vi "imageAverage.vi"(0 "Camera in":refnum<class "Camera.lvclass">, 5 "data_format":T2(ring)=enum."Mono16", 7 "roi":cluster{"x0":u64, "y0":u64, "x1":u64, "y1":u64}={"x0"=18446744073709551615, "y0"=18446744073709551615, "x1"=18446744073709551615, "y1"=18446744073709551615}, 11 "error in (no error)":errorcluster) -> (4 "Camera out":refnum<class "Camera.lvclass">, 6 "image (U8)":u8[][](array[numeric]), 8 "image (U32)":u32[][](array[numeric]), 10 "image (U64)":T1(array[cluster]), 14 "raw_image (U16)":u16[][](array[numeric]), 15 "error out":errorcluster)   [LabVIEW 2019, in "Camera.lvclass"]
doc: "Get the averaged image. This image is calculated from all recorded images in the buffer.\nThe type of the image is 2D array of pixel values. \n\nThis array is shaped depending on the resolution and ROI of the image."
uses:
  Camera.lvclass
  pco.recorder/Recorder.lvlib
  pco.convert/Convert.lvlib
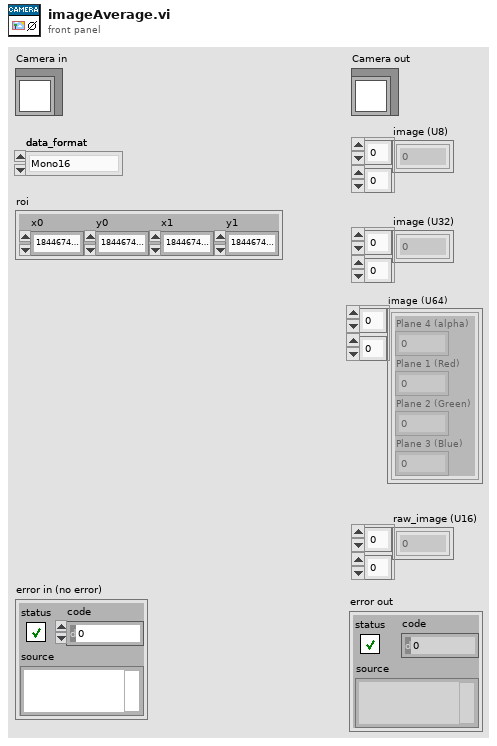
[diagram p1: front panel]
types:
  T1 = cluster{"Plane 4 (alpha)":u16, "Plane 1 (Red)":u16, "Plane 2 (Green)":u16, "Plane 3 (Blue)":u16}[][]
  T2 = enum16{"Undefined", "Mono8", "Mono16", "BGRA8", "RGBA8", "BGRA16", "RGBA16", "CompressedMono8"}
  T3 = map{enum16{"Undefined", "Mono8", "Mono16", "BGRA8", "RGBA8", "BGRA16", "RGBA16", "CompressedMono8"}, cluster{"sharpen":bool, "adaptive_sharpen":bool, "flip_vertical":bool, "auto_minmax":bool, "min_limit":u16, "max_limit":u16, "gamma":dbl, "contrast":i32, "pco_debayer_algorithm":bool, "color_temperature":i32, "color_saturation":i32, "color_vibrance":i32, "color_tint":i32, "lut_file":path}}
  T4 = map{enum16{"Undefined", "Mono8", "Mono16", "BGRA8", "RGBA8", "BGRA16", "RGBA16", "CompressedMono8"}, bool}
  T5 = cluster{"sharpen":bool, "adaptive_sharpen":bool, "flip_vertical":bool, "auto_minmax":bool, "min_limit":u16, "max_limit":u16, "gamma":dbl, "contrast":i32, "pco_debayer_algorithm":bool, "color_temperature":i32, "color_saturation":i32, "color_vibrance":i32, "color_tint":i32, "lut_file":path}
  T6 = map{enum16{"Undefined", "Mono8", "Mono16", "BGRA8", "RGBA8", "BGRA16", "RGBA16", "CompressedMono8"}, u64}
  T7 = cluster{"Blue":u16, "Green":u16, "Red":u16, "Alpha":u16}[][]
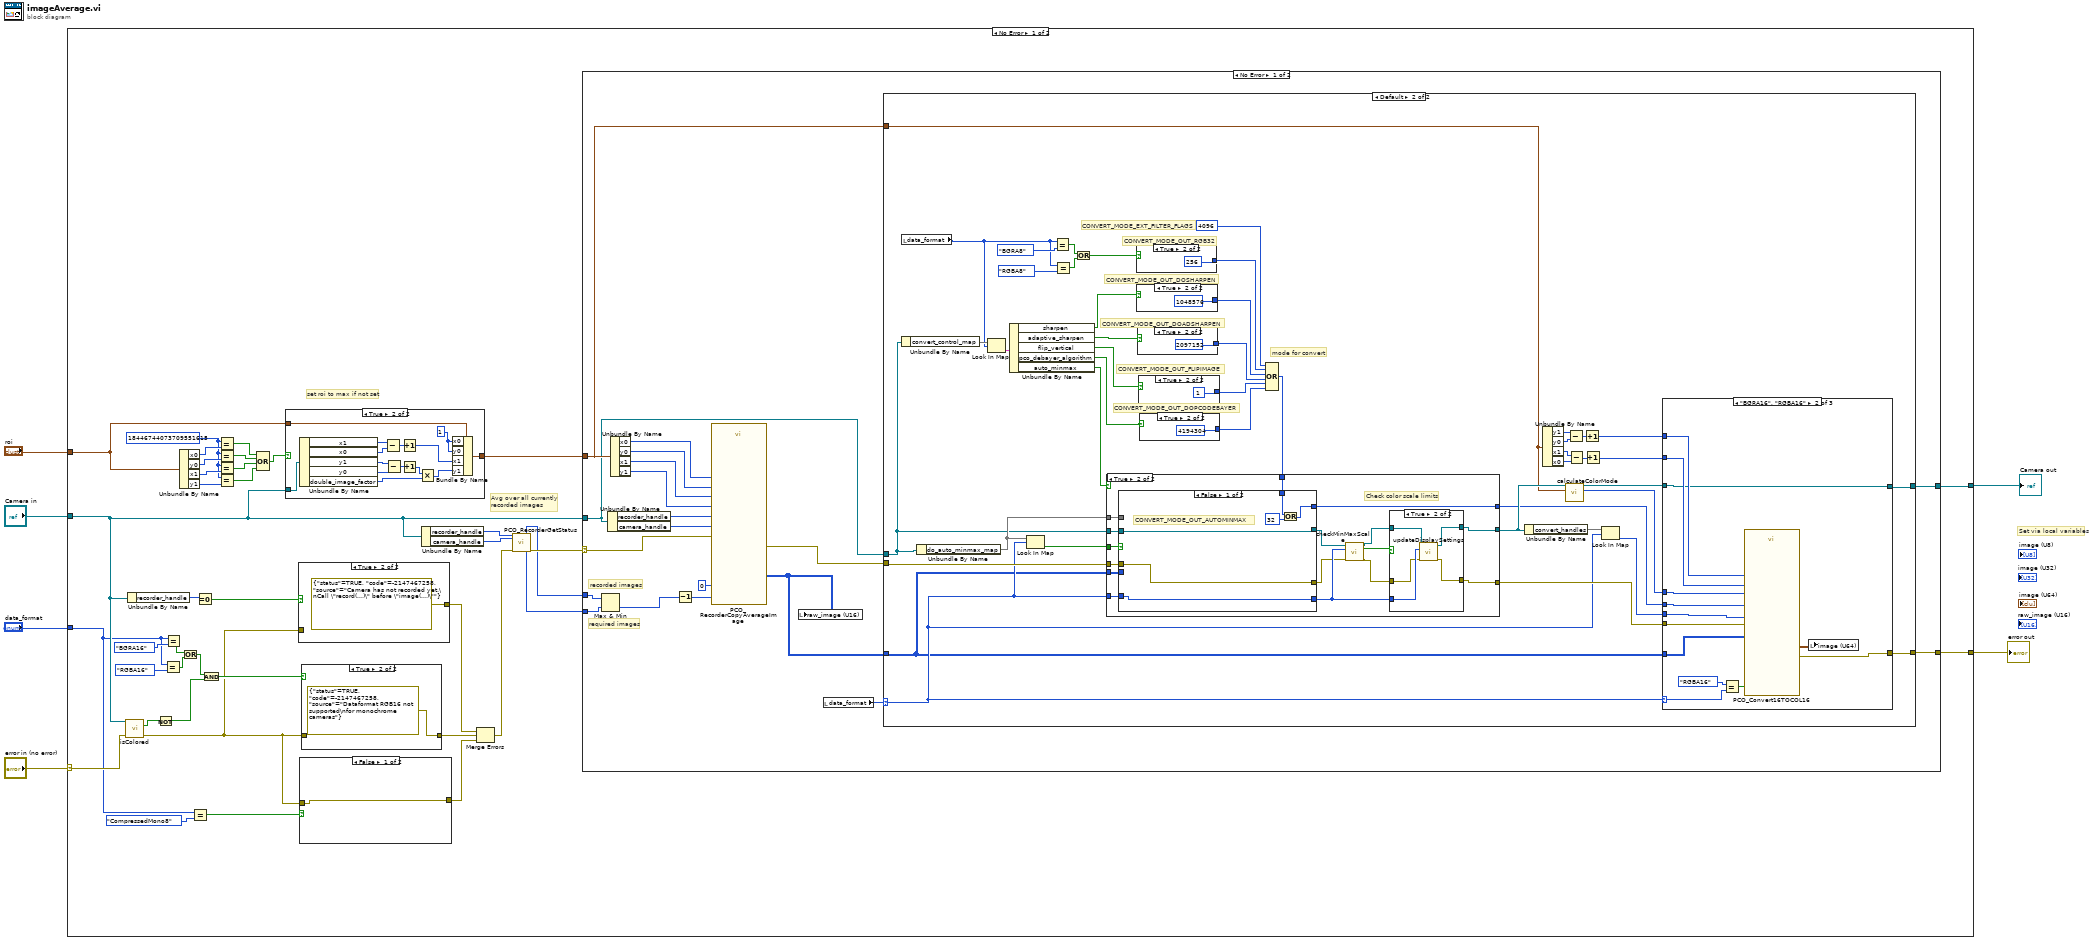
[diagram p0: block diagram]
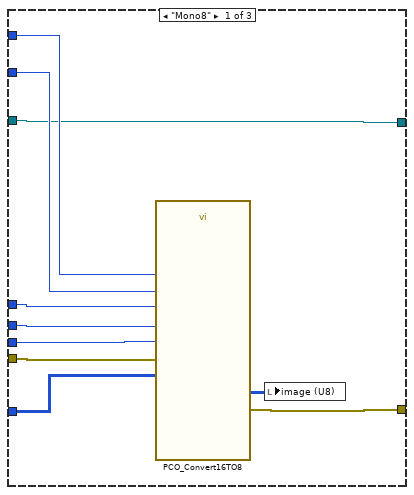
[diagram p3: hidden frame]
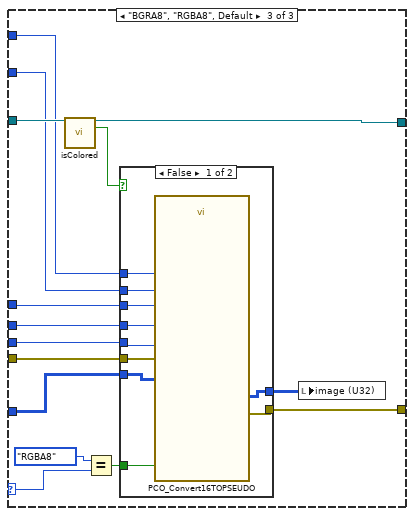
[diagram p4: hidden frame]
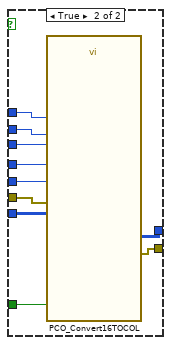
[diagram p5: hidden frame]
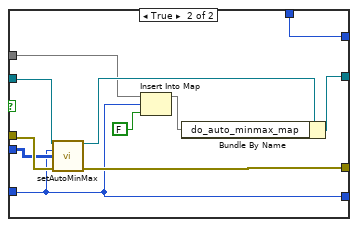
[diagram p8: hidden frame]
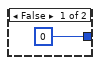
[diagram p9: hidden frame]
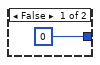
[diagram p10: hidden frame]
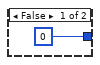
[diagram p11: hidden frame]
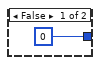
[diagram p12: hidden frame]
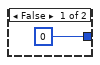
[diagram p13: hidden frame]
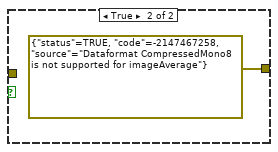
[diagram p18: hidden frame]
diagram:
  # "Set via local variables"
  n1 = case shown="No Error" "error in (no error)" {
    selector: "error in (no error)" -> [w15 w246]
    tunnel: [w23 w246] -> w3
    tunnel: [w24 w245] -> w2
    tunnel: "Camera in" -> [w22 w245]
    tunnel: "data_format" -> [w11 _]
    tunnel: "roi" -> [w26 _]
    frame No Error {
      w28 = u64 18446744073709551615 ("x0")
      # "Avg over all currently\nrecorded images"
      # "set roi to max if not set"
      n2 = call-dynamic "isColored.vi"("Camera in"=w22, "error in (no error)"=w15) -> ("colored"=w45:bool, "error out"=w40:errorcluster)  [unwired: 11 in, 1 out]
      n3 = Unbundle By Name(w22) -> ("recorder_handle"=w42:u64)
      n4 = Not(x=w45) -> (.not. x?=w44:bool)
      n5 = Equal?(x=w11, y=T2."RGBA16" ("data_format")) -> (x = y?=w10:bool)
      n6 = Equal?(x=w11, y=T2."BGRA16" ("data_format")) -> (x = y?=w9:bool)
      n7 = Unbundle By Name(w26) -> ("x0"=w32:u64, "y0"=w31:u64, "x1"=w30:u64, "y1"=w29:u64)
      n8 = Or(x=w9, y=w10) -> (x .or. y?=w8:bool)
      n9 = Equal?(x=w11, y=T2."CompressedMono8" ("data_format")) -> (x = y?=w14:bool)
      n10 = Equal To 0?(x=w42) -> (x = 0?=w41:bool)
      n11 = And(x=w8, y=w44) -> (x .and. y?=w43:bool)
      n12 = Equal?(x=w28, y=w32) -> (x = y?=w33:bool)
      n13 = Equal?(x=w28, y=w31) -> (x = y?=w34:bool)
      n14 = Equal?(x=w28, y=w30) -> (x = y?=w35:bool)
      n15 = Equal?(x=w28, y=w29) -> (x = y?=w36:bool)
      n16 = Compound Arithmetic op=OR(w33, w34, w35, w36) -> (w27:bool)
      n17 = case shown="True" w27 {
        tunnel: w22 -> [_ w238]
        tunnel: w26 -> [w224 w237]
        tunnel: [w224 w236] -> w25
        frame False {
        }
        frame True {
          w235 = u16 1 ("x0")
          n18 = Unbundle By Name(w238) -> ("x1"=w234:u64, "x0"=w233:u64, "y1"=w231:u64, "y0"=w230:u64, "double_image_factor"=w226:u16)
          n19 = Subtract(x=w234, y=w233) -> (x-y=w232:u64)
          n20 = Subtract(x=w231, y=w230) -> (x-y=w228:u64)
          n21 = Increment(x=w232) -> (x+1=w229:u64)
          n22 = Increment(x=w228) -> (x+1=w227:u64)
          n23 = Multiply(x=w227, y=w226) -> (x*y=w225:u64)
          n24 = Bundle By Name(cluster=w237, "x0"=w235, "y0"=w235, "x1"=w229, "y1"=w225) -> (w236:cluster{"x0":u64, "y0":u64, "x1":u64, "y1":u64})
        }
      }
      n25 = case shown="True" w41 {
        tunnel: w40 -> [w239 _]
        tunnel: [w239 errorcluster {"status"=TRUE, "code"=-2147467258, "source"="Camera has not recorded yet.\nCall \"record(...)\" before \"image(...)\""} ("error constant")] -> w39
        frame False {
        }
        frame True {
        }
      }
      n26 = case shown="False" w14 {
        tunnel: [w243 errorcluster {"status"=TRUE, "code"=-2147467258, "source"="Dataformat CompressedMono8  is not supported for imageAverage"} ("error constant")] -> w37
        tunnel: w40 -> [w243 _]
        frame False {
        }
        frame True {
        }
      }
      n27 = case shown="True" w43 {
        tunnel: w40 -> [w241 _]
        tunnel: [w241 errorcluster {"status"=TRUE, "code"=-2147467258, "source"="Dataformat RGB16 not supported\nfor monochrome cameras"} ("error constant")] -> w38
        frame False {
        }
        frame True {
        }
      }
      n28 = Unbundle By Name(w22) -> ("recorder_handle"=w19:u64, "camera_handle"=w18:u64)
      n29 = Merge Errors(w39, w38, w37) -> (w21:errorcluster)
      n30 = call "PCO_RecorderGetStatus.vi"("phRec"=w19, "phCam"=w18, "error in (no error)"=w21) -> ("dwProcImgCount"=w17:u32, "dwReqImgCount"=w16:u32, "error out"=w20:errorcluster)  [unwired: 5 in, 9 out]
      n31 = case shown="No Error" w20 {
        selector: w20 -> [w58 w223]
        tunnel: w25 -> [w54 _]
        tunnel: w22 -> [w50 w222]
        tunnel: [w53 w222] -> w24
        tunnel: [w52 w223] -> w23
        tunnel: w17 -> [w49 _]
        tunnel: w16 -> [w48 _]
        frame No Error {
          # "required images"
          # "recorded images"
          n32 = Max & Min(x=w49, y=w48) -> (min(x,y)=w46:u32)  [unwired: 1 out]
          n33 = Unbundle By Name(w50) -> ("recorder_handle"=w63:u64, "camera_handle"=w64:u64)
          n34 = Unbundle By Name(w54) -> ("x0"=w59:u64, "y0"=w60:u64, "x1"=w61:u64, "y1"=w62:u64)
          n35 = Decrement(x=w46) -> (x-1=w47:u32)
          n36 = call "PCO_RecorderCopyAverageImage.vi"("phRec"=w63, "wRoiX0"=w59, "wRoiX1"=w61, "phCam"=w64, "dwStartIdx"=u32 0, "dwStopIdx"=w47, "error in (no error)"=w58, "wRoiY0"=w60, "wRoiY1"=w62) -> ("wImgBuf"=w57:u16[][], "error out"=w56:errorcluster)  [unwired: 3 in, 2 out]
          n37 = local write "raw_image (U16)"(w57) -> ()
          n38 = local read "data_format"() -> (w55:T2)
          n39 = case shown="Default" w55 {
            selector: w55 -> [_ w77]
            tunnel: w56 -> [w65 w110]
            tunnel: w57 -> [_ w76]
            tunnel: w50 -> [w66 w89]
            tunnel: w54 -> [_ w107]
            tunnel: [w66 w73] -> w53
            tunnel: [w65 w74] -> w52
            frame "Mono16" {
            }
            frame Default {
              # "CONVERT_MODE_OUT_RGB32"
              # "CONVERT_MODE_OUT_FLIPIMAGE"
              # "CONVERT_MODE_OUT_DOPCODEBAYER"
              # "CONVERT_MODE_OUT_DOADSHARPEN"
              # "CONVERT_MODE_OUT_DOSHARPEN"
              # "CONVERT_MODE_EXT_FILTER_FLAGS"
              # "mode for convert"
              n40 = local read "data_format"() -> (w68:T2)
              n41 = Unbundle By Name(w89) -> ("convert_control_map"=w88:T3)
              n42 = Unbundle By Name(w89) -> ("do_auto_minmax_map"=w100:T4)
              n43 = Look In Map(map=w88, key=w68) -> (value=w98:T5)  [unwired: 1 in, 1 out]
              n44 = Unbundle By Name(w98) -> ("sharpen"=w97:bool, "adaptive_sharpen"=w96:bool, "flip_vertical"=w90:bool, "pco_debayer_algorithm"=w87:bool, "auto_minmax"=w85:bool)
              n45 = Look In Map(map=w100, key=w77) -> (value=w99:bool)  [unwired: 1 in, 1 out]
              n46 = Equal?(x=w68, y=T2."BGRA8" ("data_format")) -> (x = y?=w70:bool)
              n47 = Equal?(x=w68, y=T2."RGBA8" ("data_format")) -> (x = y?=w69:bool)
              n48 = Or(x=w70, y=w69) -> (x .or. y?=w67:bool)
              n49 = case shown="True" w67 {
                tunnel: [u32 0 ("image_index") u32 256 ("image_index")] -> w91
                frame False {
                }
                frame True {
                }
              }
              n50 = case shown="True" w97 {
                tunnel: [u32 0 ("image_index") u32 1048576 ("image_index")] -> w95
                frame False {
                }
                frame True {
                }
              }
              n51 = case shown="True" w96 {
                tunnel: [u32 0 ("image_index") u32 2097152 ("image_index")] -> w94
                frame False {
                }
                frame True {
                }
              }
              n52 = case shown="True" w90 {
                tunnel: [u32 0 ("image_index") u32 1 ("image_index")] -> w93
                frame False {
                }
                frame True {
                }
              }
              n53 = case shown="True" w87 {
                tunnel: [u32 0 ("image_index") u32 4194304 ("image_index")] -> w86
                frame False {
                }
                frame True {
                }
              }
              n54 = Compound Arithmetic op=OR(u32 4096 ("image_index"), w91, w95, w94, w93, w86) -> (w84:u32)
              n55 = case shown="True" w85 {
                tunnel: w110 -> [w169 w187]
                tunnel: [w170 w179] -> w108
                tunnel: [w171 w186] -> w79
                tunnel: w76 -> [_ w185]
                tunnel: [w169 w178] -> w78
                tunnel: w77 -> [_ w184]
                tunnel: w100 -> [_ w183]
                tunnel: w99 -> [_ w182]
                tunnel: w89 -> [w170 w181]
                tunnel: w84 -> [w171 w180]
                frame False {
                }
                frame True {
                  # "Check color scale limits"
                  n56 = case shown="False" w182 {
                    tunnel: w181 -> [w197 w211]
                    tunnel: [w198 w203] -> w186
                    tunnel: w185 -> [_ w202]
                    tunnel: w184 -> [w195 w201]
                    tunnel: [w197 w209] -> w176
                    tunnel: w187 -> [w200 w208]
                    tunnel: [w200 w207] -> w175
                    tunnel: w183 -> [_ w206]
                    tunnel: w180 -> [w196 w203]
                    tunnel: [w195 w201] -> w177
                    frame False {
                      # "CONVERT_MODE_OUT_AUTOMINMAX"
                      n57 = Or(x=w196, y=u32 32 ("image_index")) -> (x .or. y?=w198:u32)
                    }
                    frame True {
                      n58 = call-dynamic "setAutoMinMax.vi"("Camera in"=w211, "data_format"=w201, "image"=w202, "error in (no error)"=w208) -> ("Camera out"=w210:refnum<class "Camera.lvclass">, "error out"=w207:errorcluster)  [unwired: 10 in]
                      n59 = Insert Into Map(map in=w206, key=w201, value=FALSE) -> (map out=w204:T4)  [unwired: 2 out]
                      n60 = Bundle By Name(cluster=w210, "do_auto_minmax_map"=w204) -> (w209:refnum<class "Camera.lvclass">)
                    }
                  }
                  n61 = call-dynamic "checkMinMaxScale.vi"("Camera in"=w176, "data_format"=w177, "error in (no error)"=w175) -> ("Camera out"=w174:refnum<class "Camera.lvclass">, "needsUpdate"=w172:bool, "error out"=w173:errorcluster)  [unwired: 10 in]
                  n62 = case shown="True" w172 {
                    tunnel: w174 -> [w189 w194]
                    tunnel: w173 -> [w188 w190]
                    tunnel: [w189 w192] -> w179
                    tunnel: [w188 w193] -> w178
                    tunnel: w177 -> [_ w191]
                    frame False {
                    }
                    frame True {
                      n63 = call-dynamic "updateDisplaySettings.vi"("Camera in"=w194, "data_format"=w191, "error in (no error)"=w190) -> ("Camera out"=w192:refnum<class "Camera.lvclass">, "error out"=w193:errorcluster)  [unwired: 11 in]
                    }
                  }
                }
              }
              n64 = Unbundle By Name(w108) -> ("convert_handles"=w109:T6)
              n65 = Unbundle By Name(w107) -> ("y1"=w105:u64, "y0"=w106:u64, "x1"=w104:u64, "x0"=w103:u64)
              n66 = call-dynamic "calculateColorMode.vi"("Camera in"=w108, "roi"=w107) -> ("Camera out"=w81:refnum<class "Camera.lvclass">, "colorMode"=w80:i32)  [unwired: 11 in, 1 out]
              n67 = Subtract(x=w105, y=w106) -> (x-y=w102:u64)
              n68 = Subtract(x=w104, y=w103) -> (x-y=w101:u64)
              n69 = Increment(x=w102) -> (x+1=w83:u64)
              n70 = Increment(x=w101) -> (x+1=w82:u64)
              n71 = Look In Map(map=w109, key=w77) -> (value=w75:u64)  [unwired: 1 in, 1 out]
              n72 = case shown="\"BGRA16\", \"RGBA16\"" w77 {
                selector: w77 -> [_ w123 w135]
                tunnel: w75 -> [w115 w128 w141]
                tunnel: w79 -> [w116 w129 w138]
                tunnel: w80 -> [w117 w130 w137]
                tunnel: w76 -> [w113 w131 w147]
                tunnel: w83 -> [w119 w133 w140]
                tunnel: w82 -> [w118 w132 w139]
                tunnel: w78 -> [w114 w127 w142]
                tunnel: w81 -> [w111 w125 w146]
                tunnel: [w111 w125 w144] -> w73
                tunnel: [w112 w126 w145] -> w74
                frame "Mono8" {
                  n73 = call "PCO_Convert16TO8.vi"("ph"=w115, "height"=w119, "mode"=w116, "icolmode"=w117, "width"=w118, "error in (no error)"=w114, "b16"=w113) -> ("b8"=w120:u8[][], "error out"=w112:errorcluster)  [unwired: 5 in, 2 out]
                  n74 = local write "image (U8)"(w120) -> ()
                }
                frame "BGRA16", "RGBA16" {
                  n75 = Equal?(x=T2."RGBA16" ("data_format"), y=w123) -> (x = y?=w122:bool)
                  n76 = call "PCO_Convert16TOCOL16.vi"("ph"=w128, "height"=w133, "swap_colors"=w122, "mode"=w129, "icolmode"=w130, "width"=w132, "error in (no error)"=w127, "raw_image(U16)"=w131) -> ("image (U64)"=w121:T7, "error out"=w126:errorcluster)  [unwired: 4 in, 2 out]
                  n77 = local write "image (U64)"(w121) -> ()
                }
                frame "BGRA8", "RGBA8", Default {
                  n78 = call-dynamic "isColored.vi"("Camera in"=w146) -> ("Camera out"=w144:refnum<class "Camera.lvclass">, "colored"=w148:bool)  [unwired: 12 in, 1 out]
                  n79 = Equal?(x=T2."RGBA8" ("data_format"), y=w135) -> (x = y?=w134:bool)
                  n80 = case shown="False" w148 {
                    tunnel: w147 -> [w156 w166]
                    tunnel: [w158 w168] -> w145
                    tunnel: [w157 w167] -> w143
                    tunnel: w142 -> [w155 w165]
                    tunnel: w141 -> [w154 w164]
                    tunnel: w140 -> [w150 w163]
                    tunnel: w139 -> [w151 w162]
                    tunnel: w138 -> [w153 w161]
                    tunnel: w137 -> [w152 w160]
                    tunnel: w134 -> [w149 w159]
                    frame False {
                      n81 = call "PCO_Convert16TOPSEUDO.vi"("ph"=w154, "height"=w150, "swap_colors"=w149, "mode"=w153, "icolmode"=w152, "width"=w151, "error in (no error)"=w155, "b16"=w156) -> ("b32"=w157:u32[][], "error out"=w158:errorcluster)  [unwired: 4 in, 2 out]
                    }
                    frame True {
                      n82 = call "PCO_Convert16TOCOL.vi"("ph"=w164, "height"=w163, "swap_colors"=w159, "mode"=w161, "icolmode"=w160, "width"=w162, "error in (no error)"=w165, "b16"=w166) -> ("b32"=w167:u32[][], "error out"=w168:errorcluster)  [unwired: 4 in, 2 out]
                    }
                  }
                  n83 = local write "image (U32)"(w143) -> ()
                }
              }
            }
          }
        }
        frame Error {
        }
      }
    }
    frame Error {
    }
  }
  "error out" <- w3
  "Camera out" <- w2
